vi "StudentScope - Print to HTML.vi"(0 "Scope graph":refnum<vi>, 1 "CH 0 Scale":refnum<vi>, 2 "CH 1 Scale":refnum<vi>, 3 "Timebase":refnum<vi>, 4 "Ch0 Amp":string, 5 "Ch1 Amp":string, 6 "C1":string, 7 "Ch0 Freq":string, 8 "C2":string, 9 "Ch1 Freq":string, 10 "dT":string, 11 "Freq Cursor":string, 12 "Acq Rate (kHz)":dbl, 13 "Power Spectrum":refnum<vi>, 19 "Tab Control 2":enum32{"Scope", "Spectrum Analyzer"}(tab)) -> ()   [LabVIEW 2015]
uses:
  <vilib>/Utility/NIReport.llb/Append Report Text (str wrap).vi
  <vilib>/printing/OpenHTMLReport.llb/Open HTML Report in Browser (Refnum).vi
  <vilib>/Utility/NIReport.llb/NI_report.lvclass
  <vilib>/Utility/NIReport.llb/NI_ReportGenerationCore.lvlib
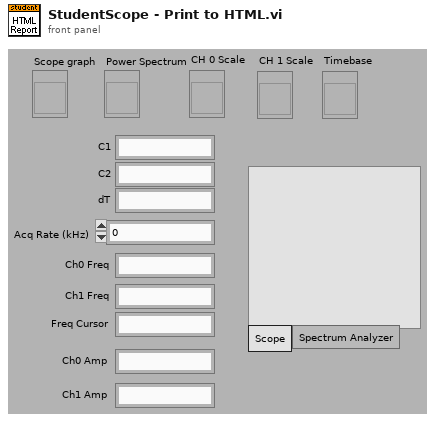
[diagram p1: front panel]
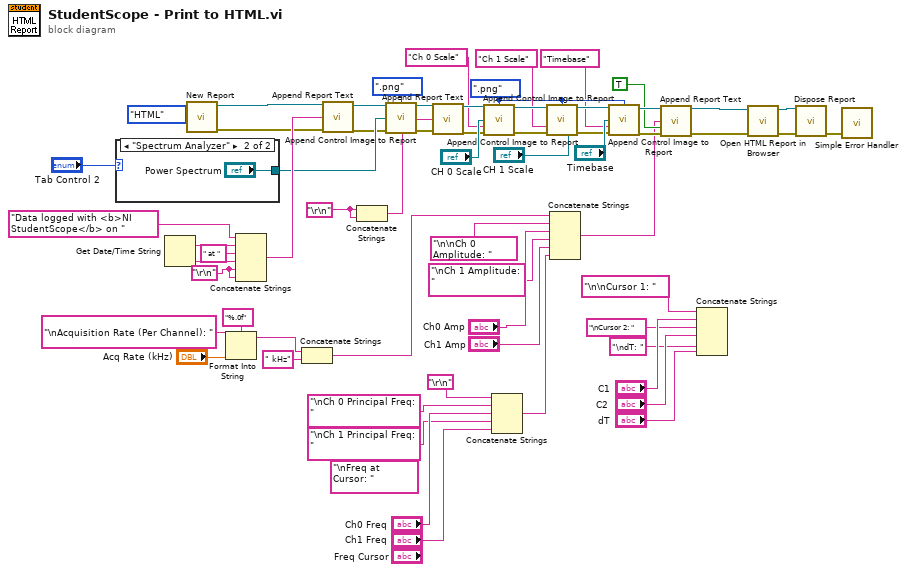
[diagram p0: block diagram]
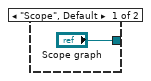
[diagram p2: hidden frame]
diagram:
  w20 = enum16{".jpg", ".png"}.".png" ("image file type(.jpg)")
  (unwired) "\nFreq at Cursor: " ("string")
  w50 = "\r\n"
  w51 = "\r\n"
  n1 = case shown="\"Spectrum Analyzer\"" "Tab Control 2" {
    tunnel: ["Scope graph" "Power Spectrum"] -> w34
    frame "Scope", Default {
    }
    frame "Spectrum Analyzer" {
    }
  }
  n2 = Get Date/Time String() -> (date string=w58:string, time string=w57:string)  [unwired: 3 in]
  n3 = call <vilib>:"New Report.vi"("report type"=enum16{"Standard Report", "HTML"}."HTML") -> ("report out"=w53:refnum<class "NI_report.lvclass">, "error out"=w52:errorcluster)  [unwired: 13 in]
  n4 = Format Into String(format string="%.0f", initial string="\nAcquisition Rate (Per Channel): ", "Acq Rate (kHz)") -> (resulting string=w12:string)  [unwired: 1 in, 1 out]
  n5 = Concatenate Strings("Data logged with <b>NI StudentScope</b> on " ("string"), w58, " at " ("string"), w57, w51, w51) -> (w54:string)
  n6 = Concatenate Strings(w12, " kHz" ("string")) -> (w5:string)
  n7 = call-poly <vilib>:"Append Report Text.vi"("report in"=w53, "text"=w54, "error in (no error)"=w52) -> ("report out"=w33:refnum<class "NI_report.lvclass">, "error out"=w32:errorcluster)  [unwired: 9 in, 2 out]
  n8 = Concatenate Strings(w50, w50) -> (w49:string)
  n9 = call-dynamic "Append Control Image to Report.vi"("report in"=w33, "image file type (.jpg)"=enum16{".jpg", ".png"}.".png" ("image file type(.jpg)"), "ctrl reference"=w34, "error in (no error)"=w32) -> ("report out"=w25:refnum<class "NI_report.lvclass">, "error out"=w26:errorcluster)  [unwired: 8 in, 2 out]
  n10 = call-poly <vilib>:"Append Report Text.vi"("report in"=w25, "text"=w49, "error in (no error)"=w26) -> ("report out"=w23:refnum<class "NI_report.lvclass">, "error out"=w24:errorcluster)  [unwired: 9 in, 2 out]
  n11 = call-dynamic "Append Control Image to Report.vi"("report in"=w23, "image file type (.jpg)"=w20, "ctrl reference"="CH 0 Scale", "description"="Ch 0 Scale", "error in (no error)"=w24) -> ("report out"=w28:refnum<class "NI_report.lvclass">, "error out"=w27:errorcluster)  [unwired: 7 in, 2 out]
  n12 = Concatenate Strings("\r\n", "\nCh 0 Principal Freq: " ("string"), "Ch0 Freq", "\nCh 1 Principal Freq: " ("string"), "Ch1 Freq") -> (w6:string)
  n13 = call-dynamic "Append Control Image to Report.vi"("report in"=w28, "image file type (.jpg)"=w20, "ctrl reference"="CH 1 Scale", "description"="Ch 1 Scale", "error in (no error)"=w27) -> ("report out"=w17:refnum<class "NI_report.lvclass">, "error out"=w18:errorcluster)  [unwired: 7 in, 2 out]
  n14 = Concatenate Strings(w5, "\n\nCh 0 Amplitude: " ("string"), "Ch0 Amp", "\nCh 1 Amplitude: " ("string"), "Ch1 Amp", w6) -> (w4:string)
  n15 = call-dynamic "Append Control Image to Report.vi"("report in"=w17, "image file type (.jpg)"=w20, "ctrl reference"="Timebase", "description"="Timebase", "error in (no error)"=w18) -> ("report out"=w15:refnum<class "NI_report.lvclass">, "error out"=w14:errorcluster)  [unwired: 7 in, 2 out]
  n16 = call-poly <vilib>:"Append Report Text.vi"("report in"=w15, "text"=w4, "append on new line? (F)"=TRUE, "error in (no error)"=w14) -> ("report out"=w3:refnum<class "NI_report.lvclass">, "error out"=w2:errorcluster)  [unwired: 8 in, 2 out]
  n17 = Concatenate Strings("\n\nCursor 1: " ("string"), "C1", "\nCursor 2: " ("string"), "C2", "\ndT: " ("string"), "dT") -> ()  [unwired: 1 out]
  n18 = call-poly <vilib>:"Open HTML Report in Browser.vi"("report in"=w3, "error in (no error)"=w2) -> ("report out"=w61:refnum<class "NI_report.lvclass">, "error out"=w60:errorcluster)  [unwired: 11 in, 1 out]
  n19 = call-dynamic "Dispose Report.vi"("report in"=w61, "error in (no error)"=w60) -> ("error out"=w62:errorcluster)  [unwired: 13 in]
  n20 = call <vilib>:"Simple Error Handler.vi"("error in (no error)"=w62) -> ()  [unwired: 4 in, 5 out]
